vi "benchmark-TagXnode.vi"() -> (2 "read":dbl=2.8434400558471685e-05 format="%#_6f", 3 "write":dbl=2.78111743927002e-05 format="%#_6f")   [LabVIEW 2017]
uses:
  <userlib>/NEVSTOP-Programming-Palette/Data/Tag/WriteTag/WriteTag_nevstop.xnode
  <userlib>/NEVSTOP-Programming-Palette/Data/Tag/ReadTag/ReadTag_nevstop.xnode
  <userlib>/_OpenG.lib/md5/md5.llb/MD5 Message Digest (Binary String)__ogtk.vi
panel:
  out "length":i32=1170
  out "outside":i32=499
  out "unit (ms)":cluster{dbl[]}[](graph)=[{[4.010200500488281e-05, 2.005577087402344e-05, 3.0074119567871094e-05, 3.0078887939453124e-05, 3.0078887939453124e-05, 3.0078887939453124e-05, 2.0051002502441405e-05, 3.0078887939453124e-05, 3.0078887939453124e-05, 3.0078887939453124e-05, 3.0083656311035158e-05, 2.0847320556640624e-05, 2.9277801513671874e-05, 3.0078887939453124e-05, 3.0236244201660155e-05, 3.071784973144531e-05, 2.9430389404296874e-05, 2.002716064453125e-05, 2.9959678649902343e-05, 3.0078887939453124e-05, 3.0074119567871094e-05, 3.0231475830078124e-05, 2.0260810852050782e-05, 2.987384796142578e-05, 2.9926300048828124e-05, 3.0083656311035158e-05, 3.0069351196289064e-05, 3.0231475830078124e-05, 2.005577087402344e-05, 3.0074119567871094e-05, 2.9926300048828124e-05, 3.0078887939453124e-05, 3.0083656311035158e-05, 3.0078887939453124e-05, 2.0046234130859375e-05, 3.0088424682617188e-05, 3.0074119567871094e-05, 3.0078887939453124e-05, 3.0078887939453124e-05, 3.0078887939453124e-05, 2.0051002502441405e-05, 3.0078887939453124e-05, 3.0078887939453124e-05, 3.0078887939453124e-05, 3.0074119567871094e-05, 3.0078887939453124e-05, 2.005577087402344e-05, 3.0083656311035158e-05, 3.0078887939453124e-05, 3.0069351196289064e-05, 3.0083656311035158e-05, 3.0078887939453124e-05, 3.0078887939453124e-05, 2.0046234130859375e-05, 3.0083656311035158e-05, 3.0078887939453124e-05, 3.0078887939453124e-05, 3.0078887939453124e-05, 3.0083656311035158e-05, 2.0046234130859375e-05, 3.0078887939453124e-05, 3.0078887939453124e-05, 3.0083656311035158e-05, 3.0078887939453124e-05, 3.0069351196289064e-05, 2.006053924560547e-05, 3.0078887939453124e-05, 3.0078887939453124e-05, 3.0078887939453124e-05, 3.0074119567871094e-05, 2.005577087402344e-05, 3.0078887939453124e-05, 3.0078887939453124e-05, 3.0074119567871094e-05, 3.0078887939453124e-05, 3.0088424682617188e-05, 2.0046234130859375e-05, 3.0074119567871094e-05, 3.0078887939453124e-05, 3.0078887939453124e-05, 3.0083656311035158e-05, 3.0078887939453124e-05, 2.0046234130859375e-05, 3.0078887939453124e-05, 3.0083656311035158e-05, 3.0078887939453124e-05, 3.0078887939453124e-05, 3.0231475830078124e-05, 2.0051002502441405e-05, 2.9926300048828124e-05, 3.0078887939453124e-05, 3.0078887939453124e-05, 3.0074119567871094e-05, 2.005577087402344e-05, 3.0088424682617188e-05, 3.0074119567871094e-05, 3.0078887939453124e-05, 3.0069351196289064e-05, 2.005577087402344e-05, 3.0083656311035158e-05, 3.0078887939453124e-05, 3.0078887939453124e-05, 3.0074119567871094e-05, 3.0078887939453124e-05, 2.005577087402344e-05, 3.0069351196289064e-05, 3.0088424682617188e-05, 3.0074119567871094e-05, 3.0078887939453124e-05, 3.0078887939453124e-05, 3.0083656311035158e-05, 2.005577087402344e-05, 3.0069351196289064e-05, 3.0078887939453124e-05, 3.0083656311035158e-05, 3.0078887939453124e-05, 3.0078887939453124e-05, 2.0051002502441405e-05, 3.0078887939453124e-05, 3.0078887939453124e-05, 3.0078887939453124e-05, 3.0074119567871094e-05, 3.0078887939453124e-05, 2.005577087402344e-05, 3.0078887939453124e-05, 3.0083656311035158e-05, 3.0069351196289064e-05, 3.0078887939453124e-05, 3.024101257324219e-05, 2.0046234130859375e-05, 2.9931068420410158e-05, 3.0069351196289064e-05, 3.0088424682617188e-05, 3.0074119567871094e-05, 3.0231475830078124e-05, 3.0078887939453124e-05, 2.9931068420410158e-05, 3.0069351196289064e-05, 3.0078887939453124e-05, 2.005577087402344e-05, 2.0203590393066405e-05, 2.9931068420410158e-05, 3.0069351196289064e-05, 3.0083656311035158e-05, 3.0231475830078124e-05, 3.0078887939453124e-05, 2.005577087402344e-05, 2.9921531677246094e-05, 3.0078887939453124e-05, 3.0231475830078124e-05, 3.0078887939453124e-05, 3.0083656311035158e-05, 2.0046234130859375e-05, 2.9926300048828124e-05, 3.0078887939453124e-05, 3.0083656311035158e-05, 3.0069351196289064e-05, 2.02178955078125e-05, 3.0069351196289064e-05, 2.9931068420410158e-05, 3.0078887939453124e-05, 3.0074119567871094e-05, 3.0078887939453124e-05, 2.005577087402344e-05, 3.0078887939453124e-05, 3.0074119567871094e-05, 3.0078887939453124e-05, 3.0078887939453124e-05, 3.0078887939453124e-05, 3.0083656311035158e-05, 2.0046234130859375e-05, 3.0088424682617188e-05, 3.0069351196289064e-05, 3.0083656311035158e-05, 3.0078887939453124e-05, 3.0078887939453124e-05, 3.0074119567871094e-05, 2.005577087402344e-05, 3.0078887939453124e-05, 3.0078887939453124e-05, 3.0074119567871094e-05, 3.0078887939453124e-05, 3.0078887939453124e-05, 3.0078887939453124e-05, 2.005577087402344e-05, 3.0074119567871094e-05, 3.0078887939453124e-05, 3.0078887939453124e-05, 3.0083656311035158e-05, 3.0078887939453124e-05, 2.0046234130859375e-05, 3.0083656311035158e-05, 3.0078887939453124e-05, 3.0078887939453124e-05, 3.0078887939453124e-05, 3.0078887939453124e-05, 2.0051002502441405e-05, 3.0078887939453124e-05, 3.0231475830078124e-05, 3.0078887939453124e-05, 2.9931068420410158e-05, 3.0069351196289064e-05, 2.0847320556640624e-05, 2.944469451904297e-05, 3.0078887939453124e-05, 3.0069351196289064e-05, 2.9935836791992188e-05, 2.0203590393066405e-05, 3.071784973144531e-05, 2.9430389404296874e-05, 3.072261810302735e-05, 2.943992614746094e-05, 3.0078887939453124e-05, 2.005577087402344e-05, 3.0078887939453124e-05, 3.0074119567871094e-05, 3.0078887939453124e-05, 3.0078887939453124e-05, 3.0083656311035158e-05, 2.005577087402344e-05, 3.0069351196289064e-05, 3.072261810302735e-05, 2.943992614746094e-05, 3.0088424682617188e-05, 2.0046234130859375e-05, 3.0074119567871094e-05, 3.0078887939453124e-05, 3.0078887939453124e-05, 3.0078887939453124e-05, 3.0078887939453124e-05, 2.0051002502441405e-05, 3.0078887939453124e-05, 3.0078887939453124e-05, 3.0083656311035158e-05, 3.070831298828125e-05, 2.9449462890625e-05, 3.0078887939453124e-05, 2.0051002502441405e-05, 3.071784973144531e-05, 2.943992614746094e-05, 3.0074119567871094e-05, 3.0078887939453124e-05, 3.070354461669922e-05, 1.9431114196777344e-05, 3.0074119567871094e-05, 3.0078887939453124e-05, 3.0078887939453124e-05, 3.0112266540527343e-05, 3.005027770996094e-05, 2.005577087402344e-05, 3.0069351196289064e-05, 3.0078887939453124e-05, 3.0083656311035158e-05, 3.0078887939453124e-05, 3.0078887939453124e-05, 2.0051002502441405e-05, 3.0078887939453124e-05, 3.0078887939453124e-05, 3.0074119567871094e-05, 3.0083656311035158e-05, 3.0074119567871094e-05, 2.005577087402344e-05, 3.0078887939453124e-05, 3.0074119567871094e-05, 3.0078887939453124e-05, 3.0078887939453124e-05, 3.072261810302735e-05, 1.941680908203125e-05, 3.070831298828125e-05, 2.943992614746094e-05, 3.0083656311035158e-05, 3.0078887939453124e-05, 3.0078887939453124e-05, 2.0046234130859375e-05, 3.0083656311035158e-05, 3.0078887939453124e-05, 3.0078887939453124e-05, 3.0078887939453124e-05, 2.0051002502441405e-05, 3.071784973144531e-05, 2.943992614746094e-05, 3.0078887939453124e-05, 3.0083656311035158e-05, 3.0078887939453124e-05, 2.0046234130859375e-05, 3.0083656311035158e-05, 3.0078887939453124e-05, 3.0069351196289064e-05, 2.9935836791992188e-05, 3.0074119567871094e-05, 3.0078887939453124e-05, 2.0051002502441405e-05, 3.0231475830078124e-05, 3.0078887939453124e-05, 2.9926300048828124e-05, 3.0088424682617188e-05, 3.0074119567871094e-05, 3.0078887939453124e-05, 2.020835876464844e-05, 3.0069351196289064e-05, 2.9931068420410158e-05, 3.0078887939453124e-05, 3.0078887939453124e-05, 3.0074119567871094e-05, 3.0078887939453124e-05, 3.0078887939453124e-05, 2.0051002502441405e-05, 3.0078887939453124e-05, 3.0078887939453124e-05, 3.0078887939453124e-05, 3.0083656311035158e-05, 3.0078887939453124e-05, 3.0069351196289064e-05, 2.005577087402344e-05, 3.0083656311035158e-05, 3.0078887939453124e-05, 3.0078887939453124e-05, 3.0074119567871094e-05, 3.0078887939453124e-05, 2.005577087402344e-05, 3.0078887939453124e-05, 3.0074119567871094e-05, 3.0078887939453124e-05, 3.0078887939453124e-05, 3.0078887939453124e-05, 2.0051002502441405e-05, 3.0078887939453124e-05, 3.024101257324219e-05, 3.0069351196289064e-05, 2.9931068420410158e-05, 2.0046234130859375e-05, 3.024101257324219e-05, 3.0112266540527343e-05, 2.9888153076171875e-05, 3.0112266540527343e-05, 3.0045509338378905e-05, 3.0078887939453124e-05, 2.0051002502441405e-05, 3.0078887939453124e-05, 3.0231475830078124e-05, 3.0078887939453124e-05, 2.9931068420410158e-05, 3.0069351196289064e-05, 2.0847320556640624e-05, 2.943992614746094e-05, 3.072261810302735e-05, 2.9430389404296874e-05, 3.0083656311035158e-05, 3.0078887939453124e-05, 2.005577087402344e-05, 3.0078887939453124e-05, 3.0074119567871094e-05, 2.9935836791992188e-05, 3.0221939086914064e-05, 3.0078887939453124e-05, 2.005577087402344e-05, 3.071308135986328e-05, 2.943992614746094e-05, 3.0112266540527343e-05, 3.005027770996094e-05, 3.071784973144531e-05, 2.943992614746094e-05, 2.0046234130859375e-05, 3.0083656311035158e-05, 2.9926300048828124e-05, 3.0231475830078124e-05, 3.0078887939453124e-05, 2.0051002502441405e-05, 3.0078887939453124e-05, 3.071784973144531e-05, 2.943992614746094e-05, 3.0074119567871094e-05, 3.0078887939453124e-05, 2.0694732666015624e-05, 2.9435157775878905e-05, 3.0078887939453124e-05, 3.0088424682617188e-05, 3.0074119567871094e-05, 3.0078887939453124e-05, 2.0046234130859375e-05, 3.0078887939453124e-05, 3.0083656311035158e-05, 3.0078887939453124e-05, 3.0088424682617188e-05, 2.0046234130859375e-05, 3.0074119567871094e-05, 3.0078887939453124e-05, 3.0078887939453124e-05, 3.0078887939453124e-05, 3.0083656311035158e-05, 2.0046234130859375e-05, 3.0078887939453124e-05, 3.0078887939453124e-05, 3.0074119567871094e-05, 3.0078887939453124e-05, 3.0078887939453124e-05, 2.005577087402344e-05, 3.0083656311035158e-05, 3.0078887939453124e-05, 3.0088424682617188e-05, 3.006458282470703e-05, 3.0078887939453124e-05, 2.005577087402344e-05, 3.0074119567871094e-05, 3.0078887939453124e-05, 3.0078887939453124e-05, 3.0078887939453124e-05, 3.0083656311035158e-05, 3.0078887939453124e-05, 2.0046234130859375e-05, 3.0078887939453124e-05, 3.0083656311035158e-05, 3.0078887939453124e-05, 3.0078887939453124e-05, 3.0074119567871094e-05, 3.0078887939453124e-05, 2.0694732666015624e-05, 2.943992614746094e-05, 3.0078887939453124e-05, 3.0083656311035158e-05, 3.070831298828125e-05, 2.943992614746094e-05, 2.005577087402344e-05, 2.9931068420410158e-05, 3.0069351196289064e-05, 3.0231475830078124e-05, 3.0083656311035158e-05, 3.009319305419922e-05, 3.005504608154297e-05, 1.99127197265625e-05, 3.0226707458496094e-05, 3.0078887939453124e-05, 3.0078887939453124e-05, 3.072261810302735e-05, 2.928733825683594e-05, 2.0046234130859375e-05, 3.0078887939453124e-05, 3.0236244201660155e-05, 3.0069351196289064e-05, 3.025054931640625e-05, 2.9764175415039063e-05, 2.0051002502441405e-05, 3.0069351196289064e-05, 3.0088424682617188e-05, 3.0226707458496094e-05, 3.0078887939453124e-05, 2.9926300048828124e-05, 2.0051002502441405e-05, 3.0078887939453124e-05, 3.0078887939453124e-05, 3.0078887939453124e-05, 3.0231475830078124e-05, 2.9931068420410158e-05, 2.0046234130859375e-05, 3.0078887939453124e-05, 3.0083656311035158e-05, 3.0231475830078124e-05, 2.9926300048828124e-05, 2.0046234130859375e-05, 3.0083656311035158e-05, 3.0078887939453124e-05, 3.0078887939453124e-05, 3.0231475830078124e-05, 2.9921531677246094e-05, 3.0088424682617188e-05, 2.0046234130859375e-05, 3.0074119567871094e-05, 3.0078887939453124e-05, 3.0078887939453124e-05, 3.0078887939453124e-05, 3.0083656311035158e-05, 2.005577087402344e-05, 3.0069351196289064e-05, 3.0083656311035158e-05, 3.0078887939453124e-05, 3.0078887939453124e-05, 3.0078887939453124e-05, 2.0051002502441405e-05, 3.0078887939453124e-05, 3.0231475830078124e-05, 3.0078887939453124e-05, 2.9931068420410158e-05, 3.0078887939453124e-05, 2.0046234130859375e-05, 3.0078887939453124e-05, 3.0231475830078124e-05, 3.0083656311035158e-05, 2.9926300048828124e-05, 3.0074119567871094e-05, 2.0847320556640624e-05, 2.9430389404296874e-05, 2.9926300048828124e-05, 3.0083656311035158e-05, 3.0088424682617188e-05, 3.0069351196289064e-05, 2.0051002502441405e-05, 3.0078887939453124e-05, 3.0078887939453124e-05, 3.0078887939453124e-05, 3.0078887939453124e-05]}, ...(2 in all)]
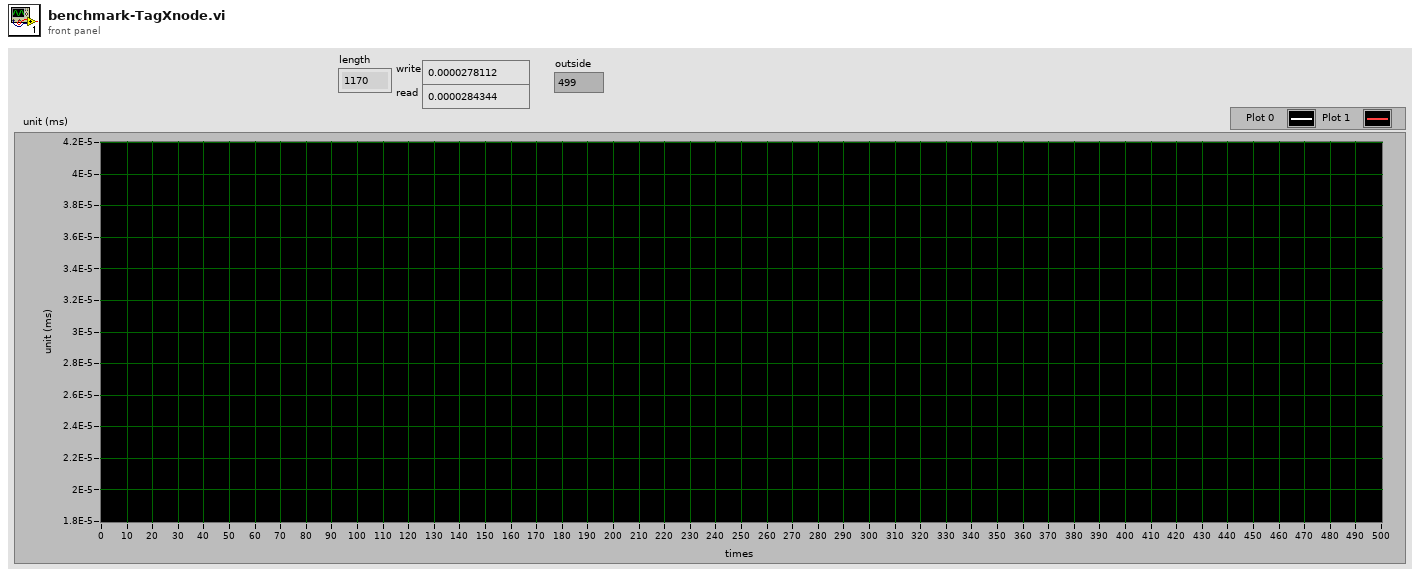
[diagram p1: front panel]
types:
  T1 = cluster{"error constant":errorcluster, "error constant 2":errorcluster, "error constant 3":errorcluster, "error constant 4":errorcluster, "error constant 5":errorcluster, "error constant 6":errorcluster, "error constant 7":errorcluster, "error constant 8":errorcluster, "error constant 9":errorcluster, "error constant 10":errorcluster, "error constant 11":errorcluster, "error constant 12":errorcluster, "error constant 13":errorcluster, "error constant 14":errorcluster, "error constant 15":errorcluster, "error constant 16":errorcluster, "error constant 17":errorcluster, "error constant 18":errorcluster, "error constant 19":errorcluster, "error constant 20":errorcluster, "error constant 21":errorcluster, "error constant 22":errorcluster, "error constant 23":errorcluster, "error constant 24":errorcluster, "error constant 25":errorcluster, "error constant 26":errorcluster, "error constant 27":errorcluster, "error constant 28":errorcluster, "error constant 29":errorcluster, "error constant 30":errorcluster, "error constant 31":errorcluster, "error constant 32":errorcluster, "error constant 33":errorcluster, "error constant 34":errorcluster, "error constant 35":errorcluster, "error constant 36":errorcluster, "error constant 37":errorcluster, "error constant 38":errorcluster, "error constant 39":errorcluster, "error constant 40":errorcluster, "error constant 41":errorcluster, "error constant 42":errorcluster, "error constant 43":errorcluster, "error constant 44":errorcluster, "error constant 45":errorcluster, "error constant 46":errorcluster, "error constant 47":errorcluster, "error constant 48":errorcluster, "error constant 49":errorcluster, "error constant 50":errorcluster, "error constant 51":errorcluster, "error constant 52":errorcluster, "error constant 53":errorcluster, "error constant 54":errorcluster, "error constant 55":errorcluster, "error constant 56":errorcluster, "error constant 57":errorcluster, "error constant 58":errorcluster, "error constant 59":errorcluster, "error constant 60":errorcluster, "error constant 61":errorcluster, "error constant 62":errorcluster, "error constant 63":errorcluster, "error constant 64":errorcluster, "error constant 65":errorcluster, cluster{"error constant":errorcluster, "error constant 2":errorcluster, "error constant 3":errorcluster, "error constant 4":errorcluster, "error constant 5":errorcluster, "error constant 6":errorcluster, "error constant 7":errorcluster, "error constant 8":errorcluster, "error constant 9":errorcluster, "error constant 10":errorcluster, "error constant 11":errorcluster, "error constant 12":errorcluster, "error constant 13":errorcluster, "error constant 14":errorcluster, "error constant 15":errorcluster, "error constant 16":errorcluster, "error constant 17":errorcluster, "error constant 18":errorcluster, "error constant 19":errorcluster, "error constant 20":errorcluster, "error constant 21":errorcluster, "error constant 22":errorcluster, "error constant 23":errorcluster, "error constant 24":errorcluster, "error constant 25":errorcluster, "error constant 26":errorcluster, "error constant 27":errorcluster, "error constant 28":errorcluster, "error constant 29":errorcluster, "error constant 30":errorcluster, "error constant 31":errorcluster, "error constant 32":errorcluster, "error constant 33":errorcluster, "error constant 34":errorcluster, "error constant 35":errorcluster, "error constant 36":errorcluster, "error constant 37":errorcluster, "error constant 38":errorcluster, "error constant 39":errorcluster, "error constant 40":errorcluster, "error constant 41":errorcluster, "error constant 42":errorcluster, "error constant 43":errorcluster, "error constant 44":errorcluster, "error constant 45":errorcluster, "error constant 46":errorcluster, "error constant 47":errorcluster, "error constant 48":errorcluster, "error constant 49":errorcluster, "error constant 50":errorcluster, "error constant 51":errorcluster, "error constant 52":errorcluster, "error constant 53":errorcluster, "error constant 54":errorcluster, "error constant 55":errorcluster, "error constant 56":errorcluster, "error constant 57":errorcluster, "error constant 58":errorcluster, "error constant 59":errorcluster, "error constant 60":errorcluster, "error constant 61":errorcluster, "error constant 62":errorcluster, "error constant 63":errorcluster, "error constant 64":errorcluster, "error constant 65":errorcluster}}
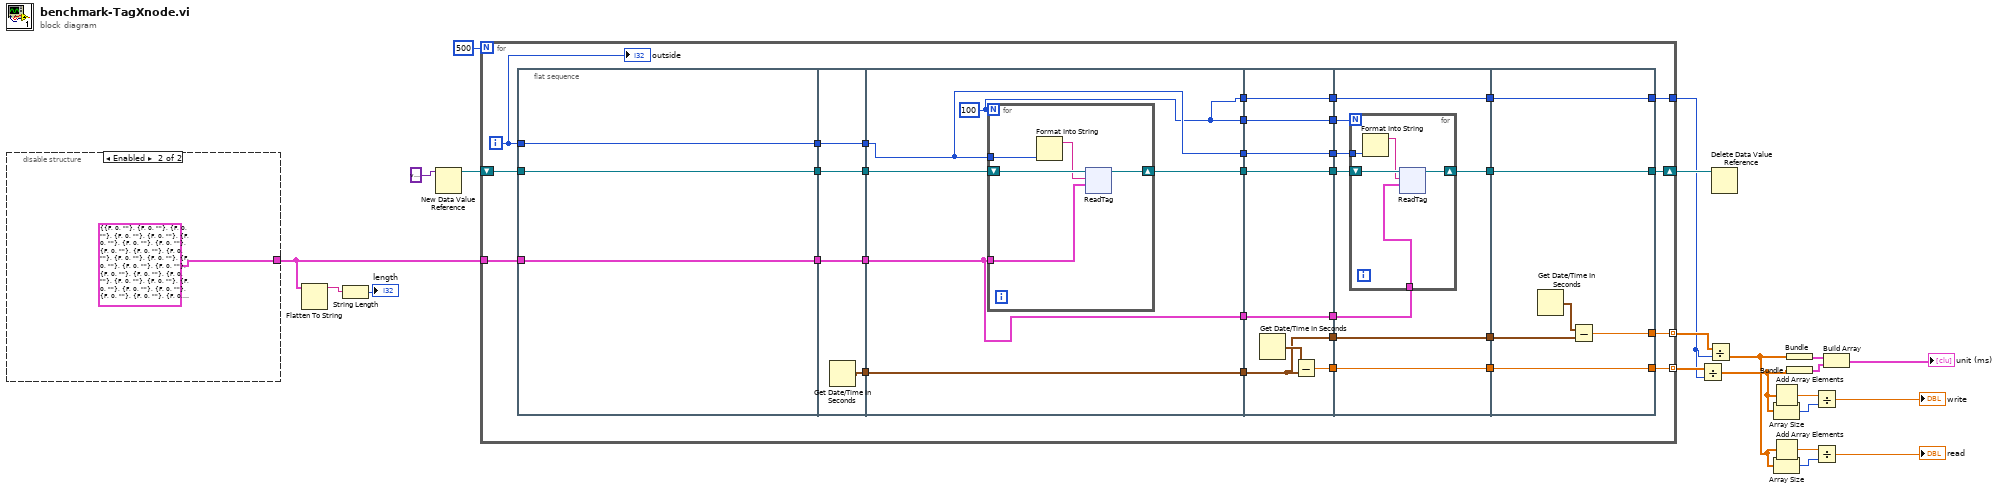
[diagram p0: block diagram]
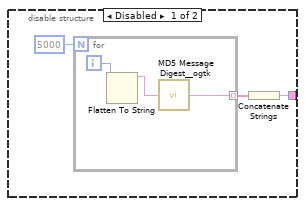
[diagram p2: hidden frame]
diagram:
  n1 = disable-structure shown="Enabled" {
    disable-tunnel: [w22 T1 {"error constant"={"status"=FALSE, "code"=0, "source"=""}, "error constant 2"={"status"=FALSE, "code"=0, "source"=""}, "error constant 3"={"status"=FALSE, "code"=0, "source"=""}, "error constant 4"={"status"=FALSE, "code"=0, "source"=""}, "error constant 5"={"status"=FALSE, "code"=0, "source"=""}, "error constant 6"={"status"=FALSE, "code"=0, "source"=""}, "error constant 7"={"status"=FALSE, "code"=0, "source"=""}, "error constant 8"={"status"=FALSE, "code"=0, "source"=""}, "error constant 9"={"status"=FALSE, "code"=0, "source"=""}, "error constant 10"={"status"=FALSE, "code"=0, "source"=""}, "error constant 11"={"status"=FALSE, "code"=0, "source"=""}, "error constant 12"={"status"=FALSE, "code"=0, "source"=""}, "error constant 13"={"status"=FALSE, "code"=0, "source"=""}, "error constant 14"={"status"=FALSE, "code"=0, "source"=""}, "error constant 15"={"status"=FALSE, "code"=0, "source"=""}, "error constant 16"={"status"=FALSE, "code"=0, "source"=""}, "error constant 17"={"status"=FALSE, "code"=0, "source"=""}, "error constant 18"={"status"=FALSE, "code"=0, "source"=""}, "error constant 19"={"status"=FALSE, "code"=0, "source"=""}, "error constant 20"={"status"=FALSE, "code"=0, "source"=""}, "error constant 21"={"status"=FALSE, "code"=0, "source"=""}, "error constant 22"={"status"=FALSE, "code"=0, "source"=""}, "error constant 23"={"status"=FALSE, "code"=0, "source"=""}, "error constant 24"={"status"=FALSE, "code"=0, "source"=""}, "error constant 25"={"status"=FALSE, "code"=0, "source"=""}, "error constant 26"={"status"=FALSE, "code"=0, "source"=""}, "error constant 27"={"status"=FALSE, "code"=0, "source"=""}, "error constant 28"={"status"=FALSE, "code"=0, "source"=""}, "error constant 29"={"status"=FALSE, "code"=0, "source"=""}, "error constant 30"={"status"=FALSE, "code"=0, "source"=""}, "error constant 31"={"status"=FALSE, "code"=0, "source"=""}, "error constant 32"={"status"=FALSE, "code"=0, "source"=""}, "error constant 33"={"status"=FALSE, "code"=0, "source"=""}, "error constant 34"={"status"=FALSE, "code"=0, "source"=""}, "error constant 35"={"status"=FALSE, "code"=0, "source"=""}, "error constant 36"={"status"=FALSE, "code"=0, "source"=""}, "error constant 37"={"status"=FALSE, "code"=0, "source"=""}, "error constant 38"={"status"=FALSE, "code"=0, "source"=""}, "error constant 39"={"status"=FALSE, "code"=0, "source"=""}, "error constant 40"={"status"=FALSE, "code"=0, "source"=""}, "error constant 41"={"status"=FALSE, "code"=0, "source"=""}, "error constant 42"={"status"=FALSE, "code"=0, "source"=""}, "error constant 43"={"status"=FALSE, "code"=0, "source"=""}, "error constant 44"={"status"=FALSE, "code"=0, "source"=""}, "error constant 45"={"status"=FALSE, "code"=0, "source"=""}, "error constant 46"={"status"=FALSE, "code"=0, "source"=""}, "error constant 47"={"status"=FALSE, "code"=0, "source"=""}, "error constant 48"={"status"=FALSE, "code"=0, "source"=""}, "error constant 49"={"status"=FALSE, "code"=0, "source"=""}, "error constant 50"={"status"=FALSE, "code"=0, "source"=""}, "error constant 51"={"status"=FALSE, "code"=0, "source"=""}, "error constant 52"={"status"=FALSE, "code"=0, "source"=""}, "error constant 53"={"status"=FALSE, "code"=0, "source"=""}, "error constant 54"={"status"=FALSE, "code"=0, "source"=""}, "error constant 55"={"status"=FALSE, "code"=0, "source"=""}, "error constant 56"={"status"=FALSE, "code"=0, "source"=""}, "error constant 57"={"status"=FALSE, "code"=0, "source"=""}, "error constant 58"={"status"=FALSE, "code"=0, "source"=""}, "error constant 59"={"status"=FALSE, "code"=0, "source"=""}, "error constant 60"={"status"=FALSE, "code"=0, "source"=""}, "error constant 61"={"status"=FALSE, "code"=0, "source"=""}, "error constant 62"={"status"=FALSE, "code"=0, "source"=""}, "error constant 63"={"status"=FALSE, "code"=0, "source"=""}, "error constant 64"={"status"=FALSE, "code"=0, "source"=""}, "error constant 65"={"status"=FALSE, "code"=0, "source"=""}, {"error constant"={"status"=FALSE, "code"=0, "source"=""}, "error constant 2"={"status"=FALSE, "code"=0, "source"=""}, "error constant 3"={"status"=FALSE, "code"=0, "source"=""}, "error constant 4"={"status"=FALSE, "code"=0, "source"=""}, "error constant 5"={"status"=FALSE, "code"=0, "source"=""}, "error constant 6"={"status"=FALSE, "code"=0, "source"=""}, "error constant 7"={"status"=FALSE, "code"=0, "source"=""}, "error constant 8"={"status"=FALSE, "code"=0, "source"=""}, "error constant 9"={"status"=FALSE, "code"=0, "source"=""}, "error constant 10"={"status"=FALSE, "code"=0, "source"=""}, "error constant 11"={"status"=FALSE, "code"=0, "source"=""}, "error constant 12"={"status"=FALSE, "code"=0, "source"=""}, "error constant 13"={"status"=FALSE, "code"=0, "source"=""}, "error constant 14"={"status"=FALSE, "code"=0, "source"=""}, "error constant 15"={"status"=FALSE, "code"=0, "source"=""}, "error constant 16"={"status"=FALSE, "code"=0, "source"=""}, "error constant 17"={"status"=FALSE, "code"=0, "source"=""}, "error constant 18"={"status"=FALSE, "code"=0, "source"=""}, "error constant 19"={"status"=FALSE, "code"=0, "source"=""}, "error constant 20"={"status"=FALSE, "code"=0, "source"=""}, "error constant 21"={"status"=FALSE, "code"=0, "source"=""}, "error constant 22"={"status"=FALSE, "code"=0, "source"=""}, "error constant 23"={"status"=FALSE, "code"=0, "source"=""}, "error constant 24"={"status"=FALSE, "code"=0, "source"=""}, "error constant 25"={"status"=FALSE, "code"=0, "source"=""}, "error constant 26"={"status"=FALSE, "code"=0, "source"=""}, "error constant 27"={"status"=FALSE, "code"=0, "source"=""}, "error constant 28"={"status"=FALSE, "code"=0, "source"=""}, "error constant 29"={"status"=FALSE, "code"=0, "source"=""}, "error constant 30"={"status"=FALSE, "code"=0, "source"=""}, "error constant 31"={"status"=FALSE, "code"=0, "source"=""}, "error constant 32"={"status"=FALSE, "code"=0, "source"=""}, "error constant 33"={"status"=FALSE, "code"=0, "source"=""}, "error constant 34"={"status"=FALSE, "code"=0, "source"=""}, "error constant 35"={"status"=FALSE, "code"=0, "source"=""}, "error constant 36"={"status"=FALSE, "code"=0, "source"=""}, "error constant 37"={"status"=FALSE, "code"=0, "source"=""}, "error constant 38"={"status"=FALSE, "code"=0, "source"=""}, "error constant 39"={"status"=FALSE, "code"=0, "source"=""}, "error constant 40"={"status"=FALSE, "code"=0, "source"=""}, "error constant 41"={"status"=FALSE, "code"=0, "source"=""}, "error constant 42"={"status"=FALSE, "code"=0, "source"=""}, "error constant 43"={"status"=FALSE, "code"=0, "source"=""}, "error constant 44"={"status"=FALSE, "code"=0, "source"=""}, "error constant 45"={"status"=FALSE, "code"=0, "source"=""}, "error constant 46"={"status"=FALSE, "code"=0, "source"=""}, "error constant 47"={"status"=FALSE, "code"=0, "source"=""}, "error constant 48"={"status"=FALSE, "code"=0, "source"=""}, "error constant 49"={"status"=FALSE, "code"=0, "source"=""}, "error constant 50"={"status"=FALSE, "code"=0, "source"=""}, "error constant 51"={"status"=FALSE, "code"=0, "source"=""}, "error constant 52"={"status"=FALSE, "code"=0, "source"=""}, "error constant 53"={"status"=FALSE, "code"=0, "source"=""}, "error constant 54"={"status"=FALSE, "code"=0, "source"=""}, "error constant 55"={"status"=FALSE, "code"=0, "source"=""}, "error constant 56"={"status"=FALSE, "code"=0, "source"=""}, "error constant 57"={"status"=FALSE, "code"=0, "source"=""}, "error constant 58"={"status"=FALSE, "code"=0, "source"=""}, "error constant 59"={"status"=FALSE, "code"=0, "source"=""}, "error constant 60"={"status"=FALSE, "code"=0, "source"=""}, "error constant 61"={"status"=FALSE, "code"=0, "source"=""}, "error constant 62"={"status"=FALSE, "code"=0, "source"=""}, "error constant 63"={"status"=FALSE, "code"=0, "source"=""}, "error constant 64"={"status"=FALSE, "code"=0, "source"=""}, "error constant 65"={"status"=FALSE, "code"=0, "source"=""}}}] -> w16
    frame Disabled {
      n2 = for {
        N: 5000 -> [_]
        tunnel: [w27] -> w24 mode=indexing
        i -> [w26]
        n3 = Flatten To String(anything=w26) -> (data string=w25:string)  [unwired: 3 in, 2 out]
        n4 = call-poly <userlib>:"MD5 Message Digest__ogtk.vi"("Message"=w25) -> ("MD5 Message Digest"=w27:string)
      }
      n5 = Concatenate Strings(w24) -> (w22:string)
    }
    frame Enabled {
    }
  }
  n6 = Flatten To String(anything=w16) -> (data string=w15:string)  [unwired: 3 in, 2 out]
  n7 = String Length(string=w15) -> (length=→"length":i32)
  n8 = New Data Value Reference(data value=variant) -> (data value reference=w18:refnum<data-value>)  [unwired: 1 in, 1 out]
  n9 = for {
    N: 500 -> [_]
    tunnel: [w57] -> w21 mode=indexing
    tunnel: [w56] -> w2
    tunnel: w16 -> [w43]
    shift-right: [w41] -> w17
    shift-left: w18 -> [w42]
    tunnel: [w36] -> w3 mode=indexing
    i -> [w54]
    n10 = flat-sequence {
      tunnel: w54 -> [w62]
      tunnel: [w60] -> w48
      tunnel: [w61] -> w46
      tunnel: [w62] -> w45
      tunnel: w43 -> [w61]
      tunnel: w42 -> [w60]
      tunnel: [w66] -> w59
      tunnel: [w65] -> w49
      tunnel: w48 -> [w65]
      tunnel: [w64] -> w47
      tunnel: w46 -> [w64]
      tunnel: w45 -> [w63]
      tunnel: [w63] -> w44
      tunnel: w59 -> [w72]
      tunnel: [w72] -> w58
      tunnel: [w68] -> w55
      tunnel: [w70] -> w50
      tunnel: w49 -> [w71]
      tunnel: w47 -> [w67]
      tunnel: w44 -> [w69]
      tunnel: [w68] -> w34
      tunnel: [w69] -> w31
      tunnel: [w67] -> w30
      tunnel: w58 -> [w104]
      tunnel: w55 -> [w106]
      tunnel: [w107] -> w53
      tunnel: [w106] -> w52
      tunnel: [w105] -> w51
      tunnel: w50 -> [w105]
      tunnel: [w104] -> w38
      tunnel: w34 -> [w103]
      tunnel: [w103] -> w33
      tunnel: [w102] -> w32
      tunnel: w31 -> [w102]
      tunnel: w30 -> [w101]
      tunnel: [w101] -> w29
      tunnel: w53 -> [w116]
      tunnel: w52 -> [w115]
      tunnel: w51 -> [w113]
      tunnel: [w116] -> w40
      tunnel: [w115] -> w39
      tunnel: w38 -> [w114]
      tunnel: [w114] -> w37
      tunnel: [w112] -> w35
      tunnel: w33 -> [w111]
      tunnel: w32 -> [w110]
      tunnel: w29 -> [w109]
      tunnel: [w155] -> w41
      tunnel: [w156] -> w56
      tunnel: [w157] -> w57
      tunnel: w40 -> [w157]
      tunnel: w39 -> [w156]
      tunnel: w37 -> [w153]
      tunnel: [w152] -> w36
      tunnel: w35 -> [w155]
      frame #0 {
      }
      frame #1 {
        n11 = Get Date/Time In Seconds() -> (seconds since 1Jan1904=w66:timestamp)
      }
      frame #2 {
        w68 = 100
        n12 = for {
          N: w68 -> [_]
          tunnel: w67 -> [w75]
          tunnel: w69 -> [w74]
          shift-right: [w76] -> w70
          shift-left: w71 -> [w77]
          n13 = Format Into String(w74) -> (resulting string=w73:string)  [unwired: 3 in, 1 out]
          n14 = xnode "ReadTag"("TagMap"=w77, "name"=w73, "Value"=w75) -> ("TagMap(dup)"=w76:refnum<data-value>)  [unwired: 1 in, 1 out]
        }
      }
      frame #3 {
        n15 = Get Date/Time In Seconds() -> (seconds since 1Jan1904=w108:timestamp)
        n16 = Subtract(x=w108, y=w104) -> (x-y=w107:dbl)
      }
      frame #4 {
        n17 = for {
          N: w111 -> [_]
          shift-right: [w120] -> w112
          shift-left: w113 -> [w121]
          tunnel: w110 -> [w118]
          tunnel: w109 -> [w117]
          n18 = Format Into String(w118) -> (resulting string=w119:string)  [unwired: 3 in, 1 out]
          n19 = xnode "ReadTag"("TagMap"=w121, "name"=w119, "Type"=w117) -> ("TagMap(dup)"=w120:refnum<data-value>)  [unwired: 1 in, 3 out]
        }
      }
      frame #5 {
        n20 = Get Date/Time In Seconds() -> (seconds since 1Jan1904=w154:timestamp)
        n21 = Subtract(x=w154, y=w153) -> (x-y=w152:dbl)
      }
    }
    "outside" <- w54
  }
  n22 = Divide(x=w21, y=w2) -> (x/y=w11:dbl[])
  n23 = Divide(x=w3, y=w2) -> (x/y=w4:dbl[])
  n24 = Delete Data Value Reference(data value reference=w17) -> ()  [unwired: 1 in, 2 out]
  n25 = Add Array Elements(numeric array=w11) -> (sum=w13:dbl)
  n26 = Array Size(array=w11) -> (size(s)=w12:i32)
  n27 = Add Array Elements(numeric array=w4) -> (sum=w6:dbl)
  n28 = Array Size(array=w4) -> (size(s)=w7:i32)
  n29 = Bundle(w4) -> (w10:cluster{dbl[]})  [unwired: 1 in]
  n30 = Bundle(w11) -> (w9:cluster{dbl[]})  [unwired: 1 in]
  n31 = Divide(x=w13, y=w12) -> (x/y=→"write":dbl)
  n32 = Divide(x=w6, y=w7) -> (x/y=→"read":dbl)
  n33 = Build Array(w10, w9) -> (→"unit (ms)":cluster{dbl[]}[])
